vi "exp 1.vi"() -> ()   [LabVIEW 2012]
panel:
  out "not or":bool
  out "not xr":bool
  out "not end":bool
  out "ex":bool
  out "or":bool
  out "and":bool
  in  "b":bool
  in  "x":bool
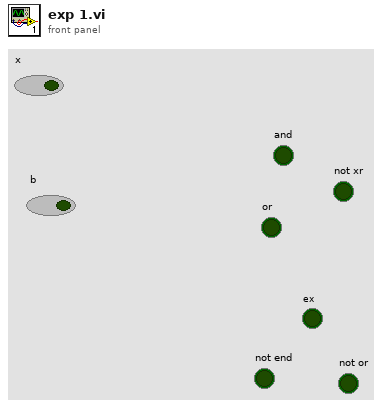
[diagram p1: front panel]
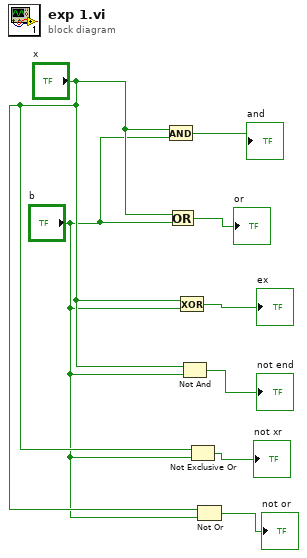
[diagram p0: block diagram]
diagram:
  n1 = And(x="x", y="b") -> (x .and. y?=→"and":bool)
  n2 = Or(x="x", y="b") -> (x .or. y?=→"or":bool)
  n3 = Exclusive Or(1:"b", 2:"x") -> (0:→"ex":bool)
  n4 = Not And(1:"b", 2:"x") -> (0:→"not end":bool)
  n5 = Not Exclusive Or(1:"b", 2:"x") -> (0:→"not xr":bool)
  n6 = Not Or(1:"b", 2:"x") -> (0:→"not or":bool)
